vi "Send Configure Arbitrary Waveform [ARB].vi"(5 "waveform handle (0)":i32, 6 "gain (1.00)":dbl=1.0 format="%.4f", 7 "Message Priority (Normal)":T1=enum."Normal", 8 "error in (no error)":errorcluster, 9 "offset (0.00 V)":dbl[unit] format="%.4f", 10 "channel name (\"CHANNEL1\")":string="CHANNEL1", 11 "Message Enqueuer":refnum<class "Message Enqueuer.lvclass">) -> (0 "error out":errorcluster, 3 "Message Enqueuer out":refnum<class "Message Enqueuer.lvclass">)   [LabVIEW 2013, in "CS++Fgen.lvlib" / "Configure Arbitrary Waveform [ARB] Msg.lvclass"]
doc: "This VI sends the message to an actor."
uses:
  Configure Arbitrary Waveform [ARB] Msg.lvclass
  <vilib>/ActorFramework/Message Enqueuer/Message Enqueuer.lvclass
  <vilib>/ActorFramework/Message Enqueuer/Message Priority.ctl
  Configure Arbitrary Waveform [ARB] Msg.lvclass/Configure Arbitrary Waveform [ARB] Msg.ctl
  <vilib>/ActorFramework/Message Enqueuer/Message Enqueuer.lvclass/Message Enqueuer.ctl
  <vilib>/ActorFramework/Message Priority Queue/Priority Enqueue.vi
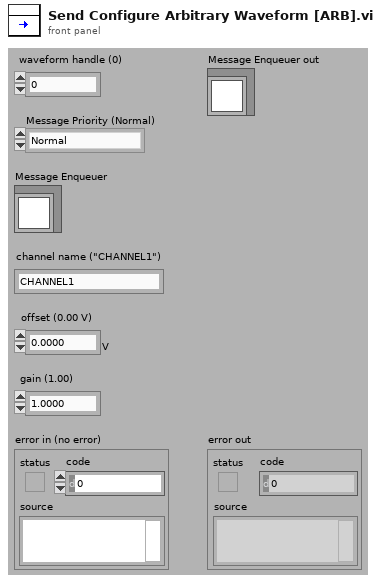
[diagram p1: front panel]
types:
  T1 = typedef "Actor Framework.lvlib/Message Enqueuer.lvclass/Message Priority.ctl" = enum16{"Low", "Normal", "High"}
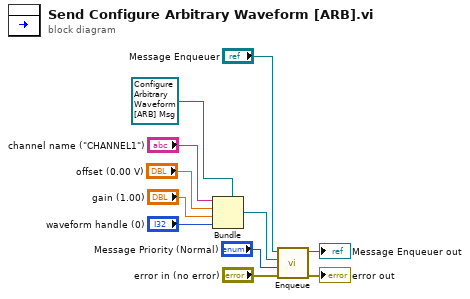
[diagram p0: block diagram]
diagram:
  n1 = Bundle(cluster=refnum<class "Configure Arbitrary Waveform [ARB] Msg.lvclass"> refnum ("Object"), "channel name (\"CHANNEL1\")", "offset (0.00 V)", "gain (1.00)", "waveform handle (0)") -> (w7:refnum<class "Configure Arbitrary Waveform [ARB] Msg.lvclass">)
  n2 = call <vilib>:"Enqueue.vi"("error in (no error)"="error in (no error)", "Message Priority (Normal)"="Message Priority (Normal)", "Message"=w7, "Message Enqueuer in"="Message Enqueuer") -> ("error out"=→"error out":errorcluster, "Message Enqueuer out"=→"Message Enqueuer out":refnum<class "Message Enqueuer.lvclass">)  [unwired: 6 in]
